vi "MSP6715-Config.vi"(8 "error in":errorcluster caption="错误输入（无错误）", 9 "等待时间(毫秒)":u32=100, 10 "恒流值":dbl, 11 "MyIndex":u8) -> (0 "error out":errorcluster)   [LabVIEW 2015, in "MSP6715.lvlib"]
uses:
  MSP6715.lvlib
  <vilib>/Instr/_visa.llb/VISA Configure Serial Port (Instr).vi
panel:
  out "VISA":refnum<visa-resource-name>
  out "返回值":u8[](array[numeric])
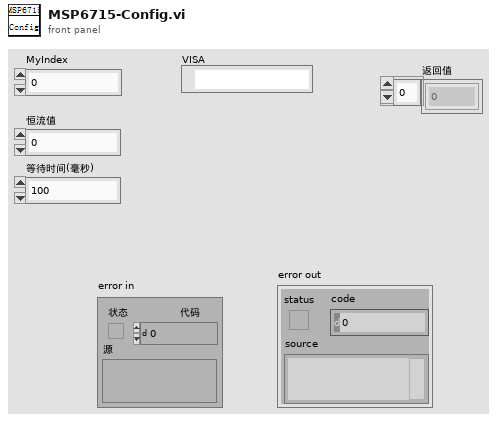
[diagram p1: front panel]
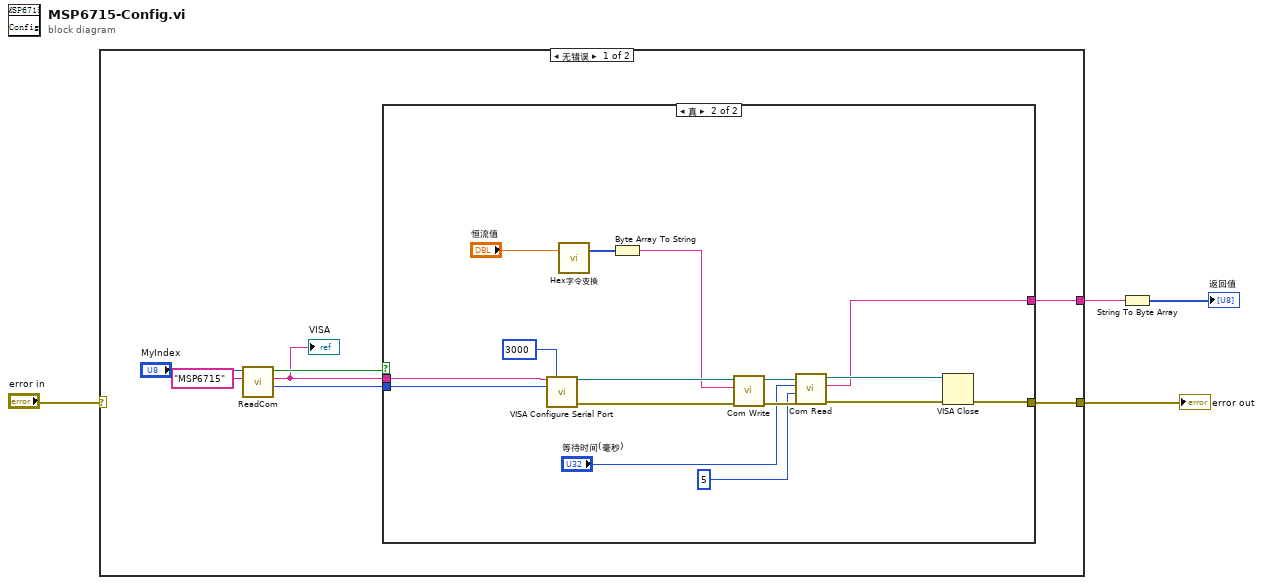
[diagram p0: block diagram]
diagram:
  n1 = case shown="无错误" "error in" {
    selector: "error in" -> [_ w28]
    tunnel: [w11 w28] -> w4
    tunnel: [w5 _] -> w2
    frame No Error {
      n2 = call "ReadCom.vi"("仪器名称"="MSP6715", "MyIndex"="MyIndex") -> ("Baudrate"=w6:i32, "COM"=w7:string, "OK?"=w8:bool)  [unwired: 7 in]
      "VISA" <- w7
      n3 = case shown="真" w8 {
        tunnel: [_ w27] -> w11
        tunnel: w7 -> [_ w26]
        tunnel: w6 -> [_ w25]
        tunnel: [_ w17] -> w5
        frame False {
        }
        frame True {
          n4 = call-poly "VISA Configure Serial Port"("VISA resource name"=w26, "timeout (10sec)"=u32 3000, "baud rate (9600)"=w25) -> ("VISA resource name out"=w23:refnum<visa-resource-name>, "error out"=w22:errorcluster)  [unwired: 11 in]
          n5 = call "Hex字令变换.vi"("数值"="恒流值") -> ("Hex指令"=w14:u32[])  [unwired: 1 in, 1 out]
          n6 = Byte Array To String(unsigned byte array=w14) -> (string=w12:string)
          n7 = call "Com Write.vi"("错误输入（无错误）"=w22, "Wbuff"=w12, "VISA In"=w23) -> ("错误输出"=w20:errorcluster, "VISA Out"=w21:refnum<visa-resource-name>)  [unwired: 7 in]
          n8 = call "Com Read.vi"("错误输入（无错误）"=w20, "num"=u32 5, "超时"="等待时间(毫秒)", "VISA In"=w21) -> ("错误输出"=w19:errorcluster, "buff"=w17:string, "VISA Out"=w18:refnum<visa-resource-name>)  [unwired: 5 in]
          n9 = VISA Close(VISA resource name=w18, error in (no error)=w19) -> (error out=w27:errorcluster)
        }
      }
    }
    frame Error {
    }
  }
  "error out" <- w4
  n10 = String To Byte Array(string=w2) -> (unsigned byte array=→"返回值":u8[])
